vi "boot up.vi"(8 "error in (no error)":errorcluster) -> (0 "error out":errorcluster, 3 "boot up":bool)   [LabVIEW 2014]
uses:
  <vilib>/CANopenLib/CANOPEN.llb/CANopen SDO Create.vi
  <vilib>/CANopenLib/CANOPEN.llb/CANopen SDO Close.vi
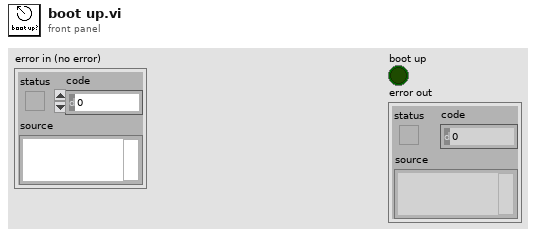
[diagram p1: front panel]
types:
  T1 = enum16{"unbekannt", "Quick stop active", "Fault reaction active", "Fault", "Operation enabled", "Switched on", "Ready to switch on", "Switch on disabled", "Not Ready to switch on"}
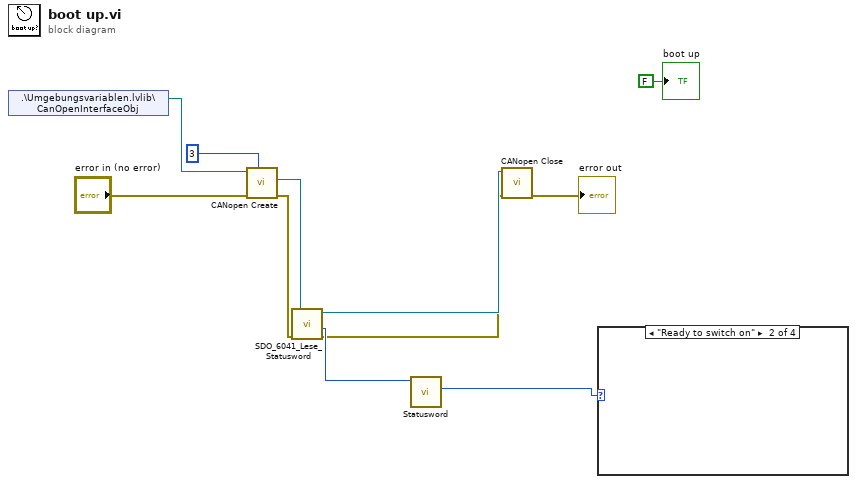
[diagram p0: block diagram]
diagram:
  n1 = shared-variable ".\\Umgebungsvariablen.lvlib\\CanOpenInterfaceObj"() -> (w11:refnum<k20>)  [unwired: 1 in, 1 out]
  n2 = call-poly <vilib>:"CANopen Create.vi"("node-ID"=u8 3, "error in (no error)"="error in (no error)", "interface object in"=w11) -> ("error out"=w4:errorcluster, "SDO object out"=w8:refnum<k20>)  [unwired: 6 in, 1 out]
  n3 = call "SDO_6041_Lese_Statusword.vi"("error in (no error)"=w4, "SDO object in"=w8) -> ("error out"=w3:errorcluster, "U16 data"=w5:u16, "SDO object out"=w7:refnum<k20>)  [unwired: 6 in, 1 out]
  n4 = call "Statusword.vi"("Wert"=w5) -> ("Status"=w6:T1)  [unwired: 10 in]
  n5 = call-poly <vilib>:"CANopen Close.vi"("error in (no error)"=w3, "SDO object in"=w7) -> ("error out"=→"error out":errorcluster)  [unwired: 9 in]
  n6 = case shown="\"Ready to switch on\"" w6 {
    frame "unbekannt", Default {
    }
    frame "Ready to switch on" {
    }
    frame "Switch on disabled" {
    }
    frame "Not Ready to switch on" {
    }
  }
  "boot up" <- FALSE ("boot up")
